vi "TCP Wait For Specific Calibration Response.vi"(0 "TCP Connection In":refnum<k5>, 1 "Next response (t)":bool=TRUE, 5 "Expected Type":T3=enum."NONE", 7 "Expected Subtype (none)":T1, 9 "Expected Message Start (\"\":any)":string, 11 "error in":errorcluster, 12 "Timeout (250 ms)":i32=250) -> (4 "TCP Connection Out":refnum<k5>, 6 "TCP Messages":string[](array[string]), 8 "Desired Response":T2, 10 "More Pwr Reporting?":bool, 15 "error out":errorcluster)   [LabVIEW 2012]
uses:
  Controls/QCA NART Response Type.ctl
  Controls/QCA NART Message.ctl
  Controls/QCA NART Response SubType.ctl
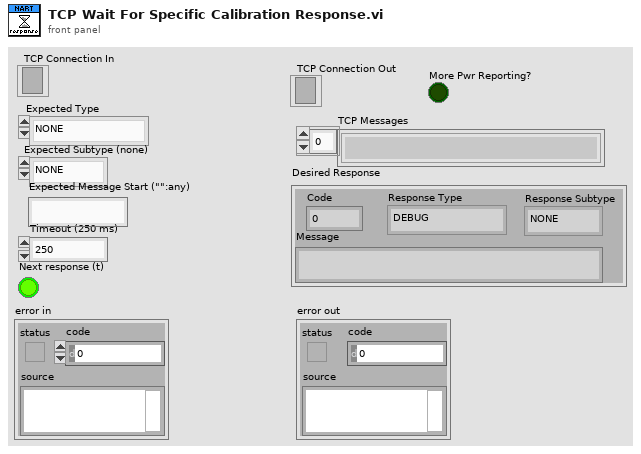
[diagram p1: front panel]
types:
  T1 = typedef "QCA NART Response SubType.ctl" = enum16{"NONE", "OK", "ON", "OFF", "BEGIN", "DONE"}
  T2 = typedef "QCA NART Message.ctl" = cluster{"Code":dbl, "Response Type":T3, "Response Subtype":T1, "Message":string}
  T3 = typedef "QCA NART Response Type.ctl" = enum16{"DEBUG", "CONTROL", "INFO", "WARNING", "ERROR", "NONE"}
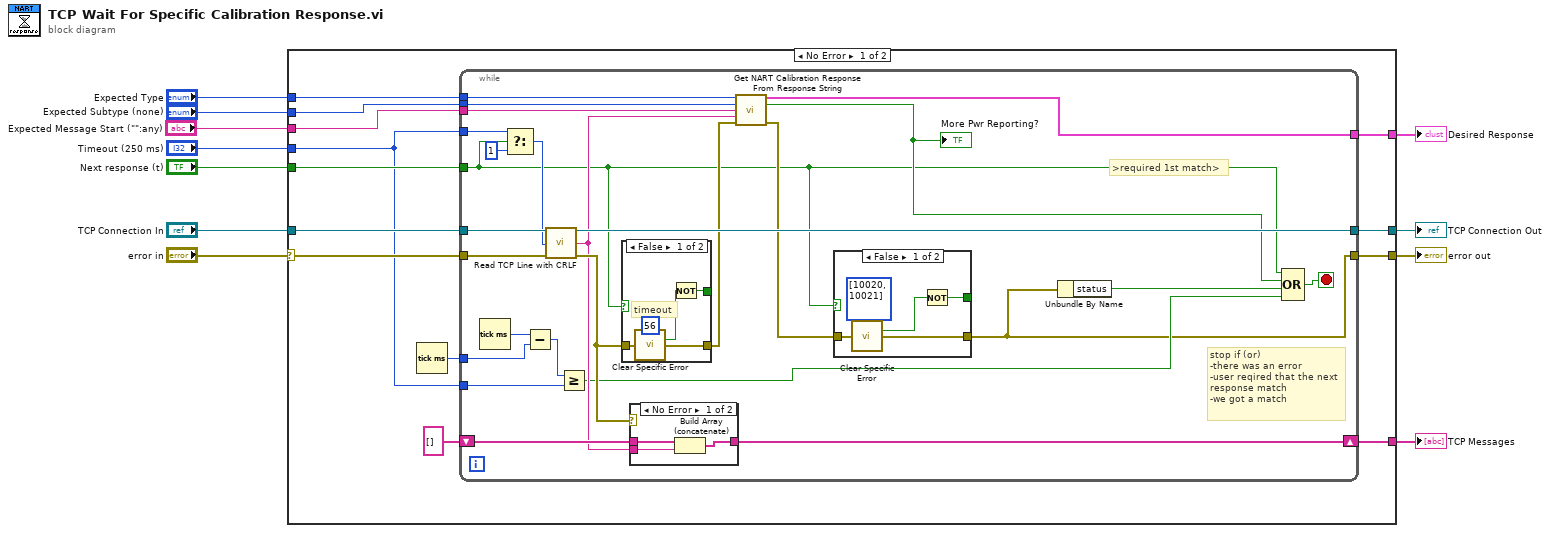
[diagram p0: block diagram]
diagram:
  n1 = case shown="No Error" "error in" {
    selector: "error in" -> [w24 w68]
    tunnel: [w15 w68] -> w8
    tunnel: "TCP Connection In" -> [w23 w67]
    tunnel: [w22 w67] -> w10
    tunnel: "Timeout (250 ms)" -> [w16 _]
    tunnel: [w19 _] -> w6
    tunnel: "Expected Type" -> [w21 _]
    tunnel: "Expected Subtype (none)" -> [w20 _]
    tunnel: "Next response (t)" -> [w18 _]
    tunnel: [w14 _] -> w2
    tunnel: "Expected Message Start (\"\":any)" -> [w12 _]
    frame No Error {
      n2 = Tick Count (ms)() -> (millisecond timer value=w17:u32)
      n3 = while {
        tunnel: w24 -> [w50]
        tunnel: w23 -> [w49]
        tunnel: [w48] -> w22
        tunnel: w21 -> [w30]
        tunnel: w20 -> [w31]
        tunnel: [w34] -> w19
        tunnel: w16 -> [w40]
        tunnel: w18 -> [w26]
        tunnel: w17 -> [w45]
        tunnel: w16 -> [w43]
        tunnel: [w25] -> w15
        shift-right: [w38] -> w14
        shift-left: string[] [] -> [w37]
        tunnel: w12 -> [w32]
        stop <- w41 stop-if-true
        # ">required 1st match>"
        # "stop if (or)\n-there was an error\n-user reqired that the next response match\n-we got a match"
        n4 = Tick Count (ms)() -> (millisecond timer value=w46:u32)
        n5 = Select(t=w40, s=w26, f=1) -> (s? t:f=w47:i32)
        n6 = Subtract(x=w46, y=w45) -> (x-y=w44:u32)
        n7 = call "Read TCP Line with CRLF.vi"("TCP Connection In"=w49, "timeout ms (100)"=w47, "error in"=w50) -> ("TCP Connection Out"=w48:refnum<k5>, "TCP Line"=w33:string, "error out"=w36:errorcluster)  [unwired: 10 in]
        n8 = Greater Or Equal?(x=w44, y=w43) -> (x >= y?=w28:bool)
        n9 = case shown="False" w26 {
          tunnel: w36 -> [w65 w66]
          tunnel: [w64 w66] -> w35
          tunnel: [w61 _] -> _
          frame False {
            # "timeout"
            n10 = call "Clear Specific Error.vi"("Specific Error Number (0: none)"=56 ("Specific Error Number"), "error in"=w65) -> ("Error Cleared?"=w62:bool, "error out"=w64:errorcluster)  [unwired: 12 in]
            n11 = Not(x=w62) -> (.not. x?=w61:bool)
          }
          frame True {
            # "1 try"
          }
        }
        n12 = case shown="No Error" w36 {
          tunnel: [w59 w60] -> w38
          tunnel: w37 -> [w58 w60]
          tunnel: w33 -> [w57 _]
          frame No Error {
            n13 = Build Array (concatenate)(w58, w57) -> (w59:string[])
          }
          frame Error {
          }
        }
        n14 = call "Get NART Calibration Response From Response String.vi"("Expected Response"=w30, "Response Subtype"=w31, "Expected Message start (\"\":any)"=w32, "TCP Line"=w33, "error in (no error)"=w35) -> ("NART Message"=w34:T2, "More Pwr Reporting?"=w29:bool, "error out"=w27:errorcluster)  [unwired: 8 in]
        "More Pwr Reporting?" <- w29
        n15 = case shown="False" w26 {
          tunnel: w27 -> [w55 w56]
          tunnel: [w54 w56] -> w25
          tunnel: [w52 _] -> _
          frame False {
            n16 = call "Clear Specific Error.vi"("Error Numbers Array (emtpy)"=i32[] [10020, 10021] ("Error Numbers Array"), "error in"=w55) -> ("Error Cleared?"=w53:bool, "error out"=w54:errorcluster)  [unwired: 12 in]
            n17 = Not(x=w53) -> (.not. x?=w52:bool)
          }
          frame True {
            # "1 try"
          }
        }
        n18 = Unbundle By Name(w25) -> ("status"=w42:bool)
        n19 = Compound Arithmetic op=OR(w26, w29, w42, w28) -> (w41:bool)
      }
    }
    frame Error {
    }
  }
  "TCP Connection Out" <- w10
  "error out" <- w8
  "Desired Response" <- w6
  "TCP Messages" <- w2
